vi "One-Motor-Speed-Control.vi"(7 "Reset":bool, 8 "Error In":errorcluster, 11 "速度(秒/度)":dbl) -> (0 "Error Out":errorcluster)   [LabVIEW 2019]
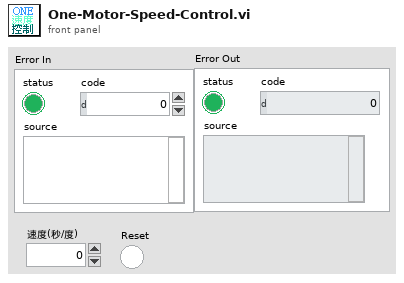
[diagram p1: front panel]
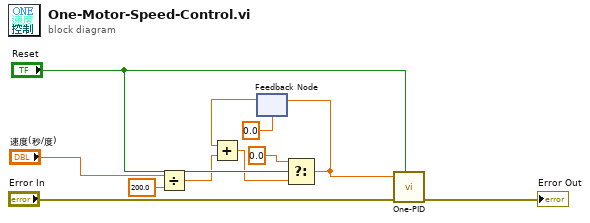
[diagram p0: block diagram]
diagram:
  n1 = Divide(x="速度(秒/度)", y=200.0) -> (x/y=w2:dbl)
  n2 = feedback #1(0.0) -> (w3:dbl)
  n3 = Add(x=w3, y=w2) -> (x+y=w1:dbl)
  n4 = Select(t=0.0, s="Reset", f=w1) -> (s? t:f=w4:dbl)
  n5 = feedback-in #1(w4) -> ()
  n6 = call "One-PID.vi"("Reset"="Reset", "Error In"="Error In", "目標角度"=w4) -> ("Error Out"=→"Error Out":errorcluster)  [unwired: 8 in]
